vi "시간..16-0329.vi"() -> ()   [LabVIEW 2014]
panel:
  in  "정지":bool
  in  "Time Target (s)":dbl=1.0 caption="타겟 시간(초)"
  out "현재 시간":timestamp
  out "ms 타이머 값":u32
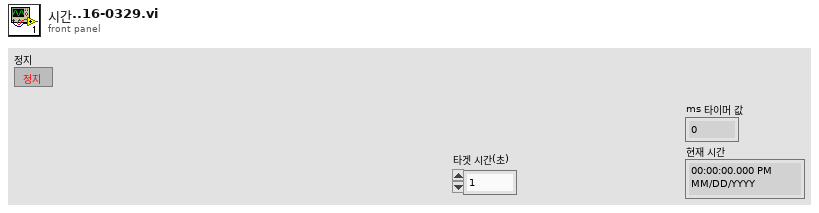
[diagram p1: front panel]
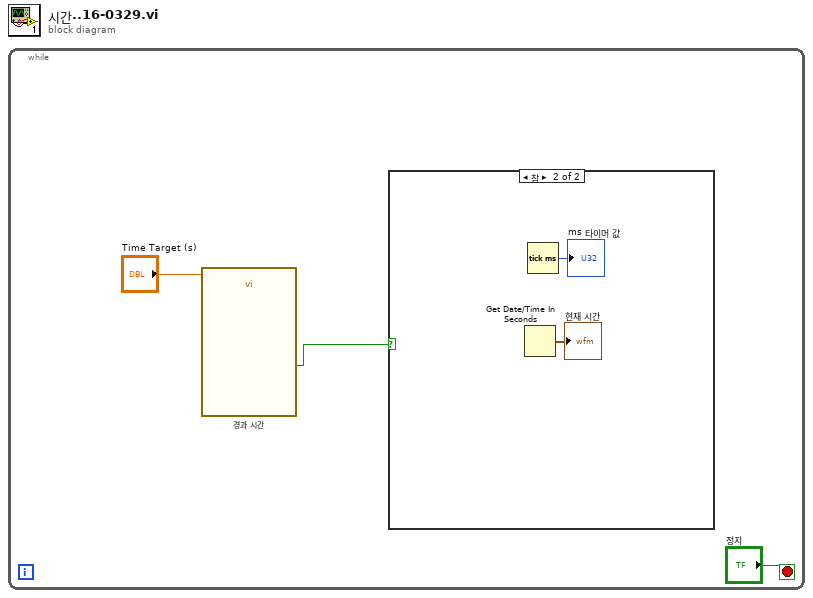
[diagram p0: block diagram]
diagram:
  n1 = while {
    stop <- "정지" stop-if-true
    n2 = call "경과 시간"("Time Target (s)"="Time Target (s)") -> ("Time has Elapsed"=w3:bool)  [unwired: 11 in, 7 out]
    n3 = case shown="참" w3 {
      frame False {
      }
      frame True {
        n4 = Get Date/Time In Seconds() -> (seconds since 1Jan1904=→"현재 시간":timestamp)
        n5 = Tick Count (ms)() -> (millisecond timer value=→"ms 타이머 값":u32)
      }
    }
  }
